vi "Parse 16-1.vi"(11 "String":string) -> (3 "Puzzle 16-1":T1)   [LabVIEW 2020]
uses:
  Puzzle 16-1.ctl
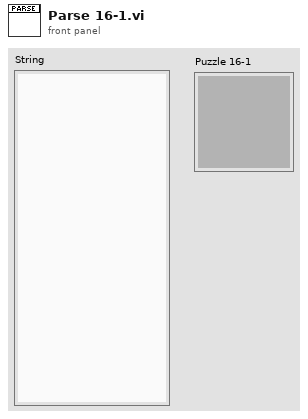
[diagram p1: front panel]
types:
  T1 = typedef "Puzzle 16-1.ctl" = cluster{}
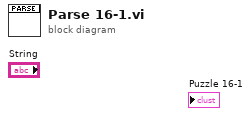
[diagram p0: block diagram]
diagram:
